vi "5-2_FanControl.vi"() -> ()   [LabVIEW 2014]
doc: "This example demonstrates how to read one channel of digital input from a LINX device.\n------------------------------------\nAuther: Koji Ohashi\nCopyright (c) 2020 Japan LabVIEW Users Group, Volunteer members.\nThis VI is released under the MIT License.\nhttp://opensource.org/licenses/mit-license.php\n------------------------------------"
uses:
  <vilib>/MakerHub/LINX/LMH-LINX.lvlib
  <vilib>/MakerHub/LINX/Public/Peripherals/Digital/Digital Read 1 Chan.vi
  <vilib>/MakerHub/LINX/Public/Utilities/Open Serial.vi
  <vilib>/MakerHub/LINX/Public/Peripherals/PWM/PWM Set Duty Cycle 1 Chan.vi
panel:
  out "Count":i32
  out "DI Value":bool
  in  "DI Channel":u8=2
  in  "Stop Button":bool
  in  "Serial Port":refnum<visa-resource-name>
  # "LINX Device Settings"
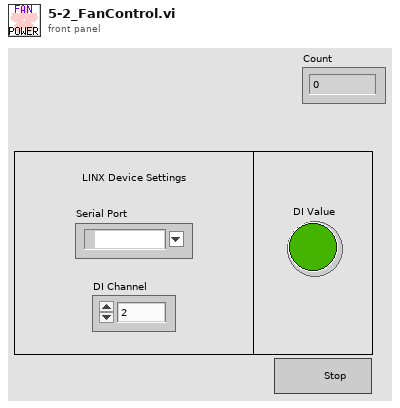
[diagram p1: front panel]
types:
  T1 = typedef "LMH-LINX.lvlib/LINX Ref.ctl" = cluster{"IO":T2, "Interface":T3, "LINX Device Config":T4}
  T2 = typedef "LMH-LINX.lvlib/Platform.ctl" = enum16{"Remote", "Local"}
  T3 = typedef "LMH-LINX.lvlib/Interface.ctl" = enum16{"Serial", "TCP"}
  T4 = typedef "LMH-LINX.lvlib/Device.lvlib/LINX Device Config.ctl" = cluster{"Interface":T3, "COM Port":refnum<visa-resource-name>, "TCP Configuration":T5, "Device Family":u8, "Device ID":u8, "Device Name":string, "TCP Ref":refnum<k5>, "Channels":T6}
  T5 = typedef "LMH-LINX.lvlib/Device.lvlib/TCP Config.ctl" = cluster{"IP Address":string, "Port":u16}
  T6 = typedef "LMH-LINX.lvlib/Channels.ctl" = cluster{"DI":u8[], "DO":u8[], "AI":u8[], "AO":u8[], "PWM":u8[], "QE":u8[], "UART":u8[], "I2C 2":u8[], "SPI":u8[], "CAN":u8[], "Servo":u8[], "AI Ref (V)":dbl, "AI Resolution (Bits)":u8, "AO Ref (V)":dbl, "AO Resolution (Bits)":u8}
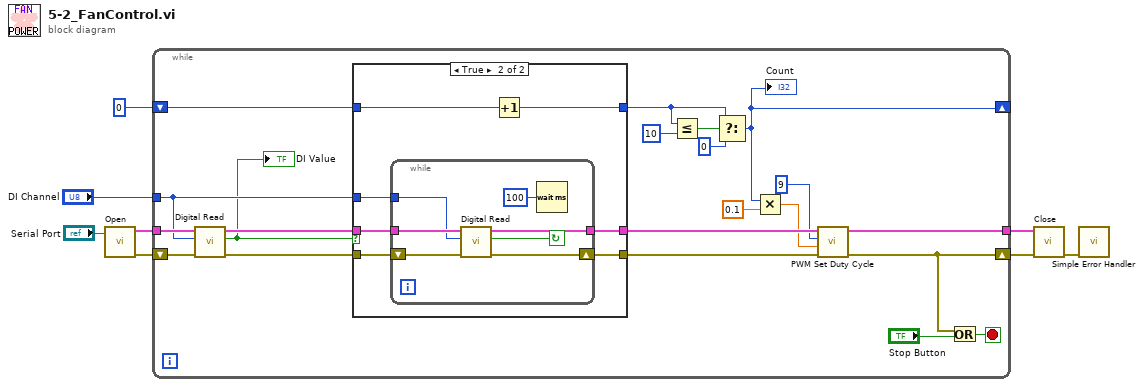
[diagram p0: block diagram]
diagram:
  n1 = call-poly <vilib>:"Open.vi"("Serial Port"="Serial Port") -> ("Error Out"=w7:errorcluster, "LINX Resource"=w8:T1)  [unwired: 8 in, 1 out]
  n2 = while {
    tunnel: w8 -> [w27]
    tunnel: [w15] -> w6
    shift-right: [w13] -> w5
    shift-left: w7 -> [w26]
    tunnel: "DI Channel" -> [w21]
    shift-right: [w10] -> _
    shift-left: 0 -> [w19]
    stop <- w29 stop-if-true
    n3 = call-poly <vilib>:"Digital Read.vi"("Error In"=w26, "DI Channel"=w21, "LINX Resource"=w27) -> ("Error Out"=w20:errorcluster, "DI Value"=w17:bool, "LINX Resource"=w22:T1)  [unwired: 6 in]
    "DI Value" <- w17
    n4 = case shown="TRUE" w17 {
      tunnel: w22 -> [w30 w39]
      tunnel: w21 -> [_ w38]
      tunnel: w20 -> [w32 w37]
      tunnel: [w32 w36] -> w14
      tunnel: w19 -> [w31 w33]
      tunnel: [w31 w35] -> w18
      tunnel: [w30 w34] -> w16
      frame False {
      }
      frame True {
        n5 = while {
          tunnel: w39 -> [w46]
          tunnel: w38 -> [w45]
          shift-right: [w43] -> w36
          shift-left: w37 -> [w44]
          tunnel: [w40] -> w34
          stop <- w41 continue-if-true
          n6 = call-poly <vilib>:"Digital Read.vi"("Error In"=w44, "DI Channel"=w45, "LINX Resource"=w46) -> ("Error Out"=w43:errorcluster, "DI Value"=w41:bool, "LINX Resource"=w40:T1)  [unwired: 6 in]
          n7 = Wait (ms)(milliseconds to wait=u32 100) -> ()  [unwired: 1 out]
        }
        n8 = Increment(x=w33) -> (x+1=w35:i32)
      }
    }
    n9 = Less Or Equal?(x=w18, y=10) -> (x <= y?=w24:bool)
    n10 = Select(t=w18, s=w24, f=0) -> (s? t:f=w10:i32)
    "Count" <- w10
    n11 = Multiply(x=w10, y=0.1) -> (x*y=w9:dbl)
    n12 = call-poly <vilib>:"PWM Set Duty Cycle.vi"("Error In"=w14, "Duty Cycle (0-1)"=w9, "PWM Channel"=u8 9, "LINX Resource"=w16) -> ("Error Out"=w13:errorcluster, "LINX Resource"=w15:T1)  [unwired: 6 in]
    n13 = Or(x=w13, y="Stop Button") -> (x .or. y?=w29:bool)
  }
  n14 = call <vilib>:"Close.vi"("Error In"=w5, "LINX Resource"=w6) -> ("Error Out"=w3:errorcluster)  [unwired: 9 in]
  n15 = call <vilib>:"Simple Error Handler.vi"("error in (no error)"=w3) -> ()  [unwired: 4 in, 5 out]
